vi "Show_Hide FP Items.vi"(8 "error in (no error)":errorcluster, 10 "active wheel types":T1={"Wheel Type"=TRUE, "X Position"=TRUE, "Y Position"=TRUE, "Frame Angle"=TRUE, "Wheel Name"=TRUE, "Wheel Radius"=TRUE, "Gear Ratio"=TRUE, "Forward Rotation Direction"=TRUE, "Steering Gear Ratio"=TRUE, "Motor Angle Offset"=TRUE, "Min Steering Angle"=TRUE, "Max Steering Angle"=TRUE, "Steering Range"=TRUE, "Caster Gear Ratio"=TRUE, "Forward Offset"=TRUE, "Roller Orientation"=TRUE}, 11 "fp refs":T2) -> (0 "error out":errorcluster)   [LabVIEW 2017, in "NI_Robotics_Configure Steering Frame.lvlib" / "User Defined Frame Subpanel.lvlib"]
uses:
  <vilib>/robotics/Dialog/Configure Steering Frame/User Defined Frame Subpanel/User Defined Frame Subpanel.lvlib
  <vilib>/robotics/Dialog/Configure Steering Frame/User Defined Frame Subpanel/FP Refs.ctl
  <vilib>/robotics/Dialog/Configure Steering Frame/User Defined Frame Subpanel/Enabled Items.ctl
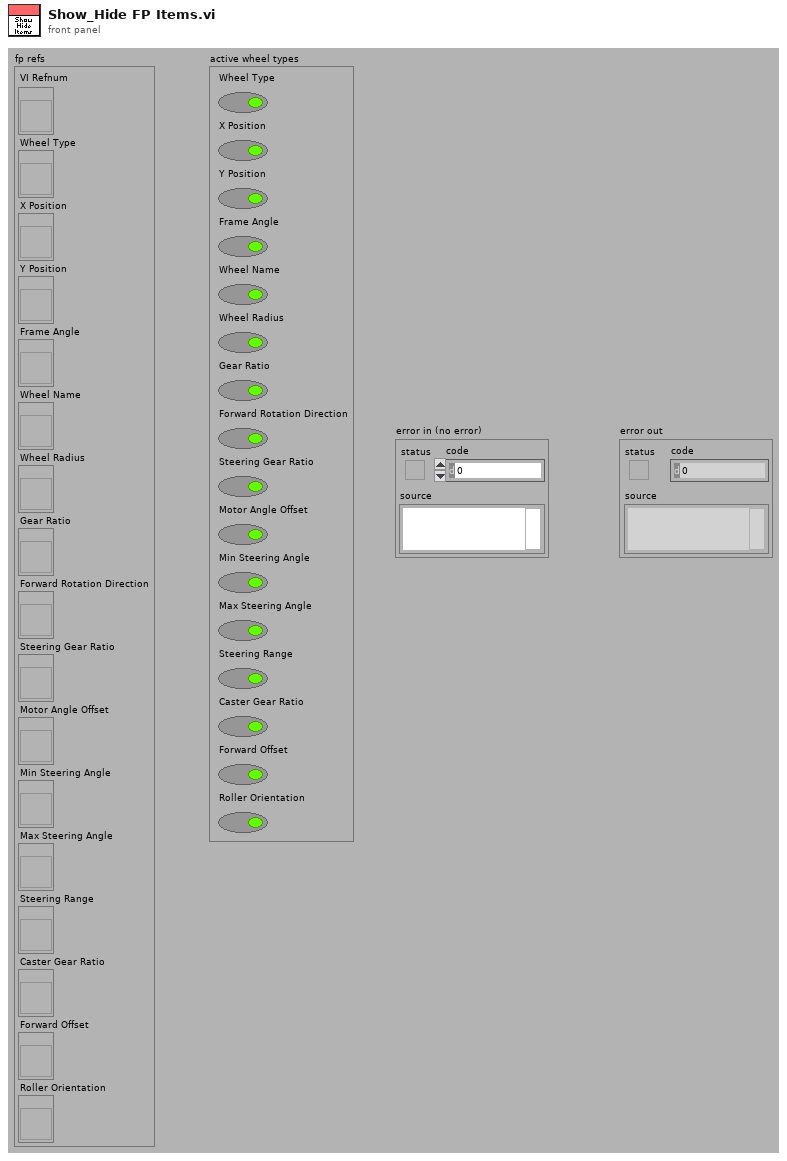
[diagram p1: front panel]
types:
  T1 = typedef "NI_Robotics_Configure Steering Frame.lvlib/User Defined Frame Subpanel.lvlib/Enabled Items.ctl" = cluster{"Wheel Type":bool, "X Position":bool, "Y Position":bool, "Frame Angle":bool, "Wheel Name":bool, "Wheel Radius":bool, "Gear Ratio":bool, "Forward Rotation Direction":bool, "Steering Gear Ratio":bool, "Motor Angle Offset":bool, "Min Steering Angle":bool, "Max Steering Angle":bool, "Steering Range":bool, "Caster Gear Ratio":bool, "Forward Offset":bool, "Roller Orientation":bool}
  T2 = typedef "NI_Robotics_Configure Steering Frame.lvlib/User Defined Frame Subpanel.lvlib/FP Refs.ctl" = cluster{"VI Refnum":refnum<vi>, "Wheel Type":refnum<vi>, "X Position":refnum<vi>, "Y Position":refnum<vi>, "Frame Angle":refnum<vi>, "Wheel Name":refnum<vi>, "Wheel Radius":refnum<vi>, "Gear Ratio":refnum<vi>, "Forward Rotation Direction":refnum<vi>, "Steering Gear Ratio":refnum<vi>, "Motor Angle Offset":refnum<vi>, "Min Steering Angle":refnum<vi>, "Max Steering Angle":refnum<vi>, "Steering Range":refnum<vi>, "Caster Gear Ratio":refnum<vi>, "Forward Offset":refnum<vi>, "Roller Orientation":refnum<vi>}
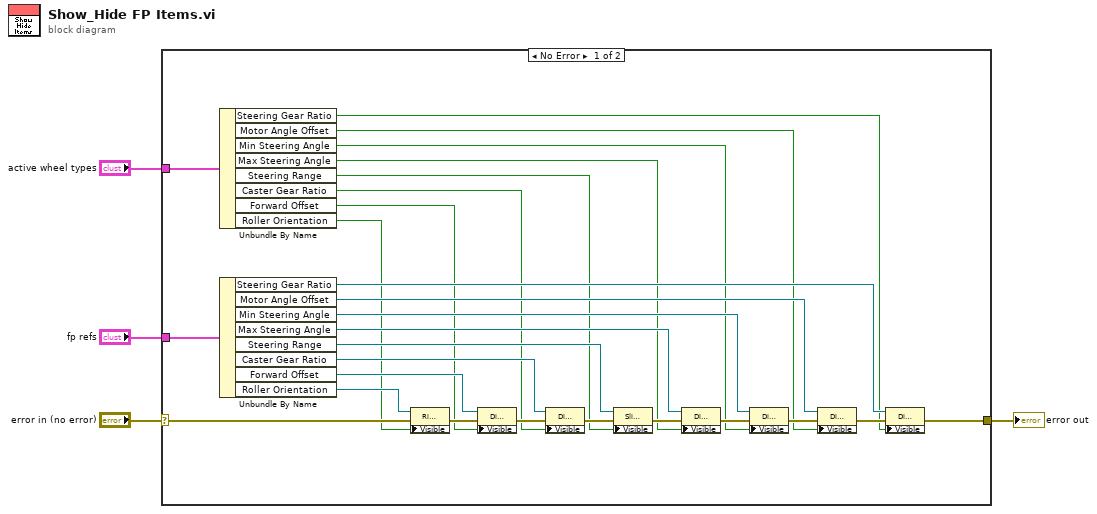
[diagram p0: block diagram]
diagram:
  n1 = case shown="No Error" "error in (no error)" {
    selector: "error in (no error)" -> [w29 w32]
    tunnel: [w14 w32] -> w3
    tunnel: "fp refs" -> [w31 _]
    tunnel: "active wheel types" -> [w13 _]
    frame No Error {
      n2 = Unbundle By Name(w13) -> ("Steering Gear Ratio"=w12:bool, "Motor Angle Offset"=w11:bool, "Min Steering Angle"=w10:bool, "Max Steering Angle"=w9:bool, "Steering Range"=w8:bool, "Caster Gear Ratio"=w7:bool, "Forward Offset"=w6:bool, "Roller Orientation"=w5:bool)
      n3 = Unbundle By Name(w31) -> ("Steering Gear Ratio"=w15:refnum<vi>, "Motor Angle Offset"=w17:refnum<vi>, "Min Steering Angle"=w19:refnum<vi>, "Max Steering Angle"=w21:refnum<vi>, "Steering Range"=w23:refnum<vi>, "Caster Gear Ratio"=w25:refnum<vi>, "Forward Offset"=w28:refnum<vi>, "Roller Orientation"=w30:refnum<vi>)
      n4 = property class="Ring (strict)"(reference=w30, error in=w29, "Visible"=w5) -> (error out=w27:errorcluster)  [unwired: 1 out]
      n5 = property class="DigNum (strict)"(reference=w28, error in=w27, "Visible"=w6) -> (error out=w26:errorcluster)  [unwired: 1 out]
      n6 = property class="DigNum (strict)"(reference=w25, error in=w26, "Visible"=w7) -> (error out=w24:errorcluster)  [unwired: 1 out]
      n7 = property class="Slide (strict)"(reference=w23, error in=w24, "Visible"=w8) -> (error out=w22:errorcluster)  [unwired: 1 out]
      n8 = property class="DigNum (strict)"(reference=w21, error in=w22, "Visible"=w9) -> (error out=w20:errorcluster)  [unwired: 1 out]
      n9 = property class="DigNum (strict)"(reference=w19, error in=w20, "Visible"=w10) -> (error out=w18:errorcluster)  [unwired: 1 out]
      n10 = property class="DigNum (strict)"(reference=w17, error in=w18, "Visible"=w11) -> (error out=w16:errorcluster)  [unwired: 1 out]
      n11 = property class="DigNum (strict)"(reference=w15, error in=w16, "Visible"=w12) -> (error out=w14:errorcluster)  [unwired: 1 out]
    }
    frame Error {
    }
  }
  "error out" <- w3
